vi "solar_log Banner Dialog.vi"() -> ()   [LabVIEW 2018]
doc: "This displays an error notification bar across the top of the primary monitor."
panel:
  in  "Close":bool
  in  "Error":string caption="Fault Summary:"
  # "ERROR"
  # "Click to Close"
  # "ERROR"
  # "Click to Close"
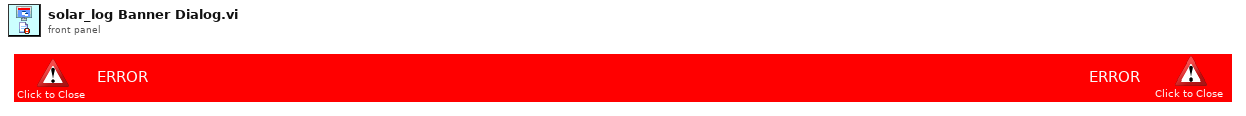
[diagram p1: front panel]
types:
  T1 = typedef "LVRectTypeDef.ctl" = cluster{"Left":i16, "Top":i16, "Right":i16, "Bottom":i16}
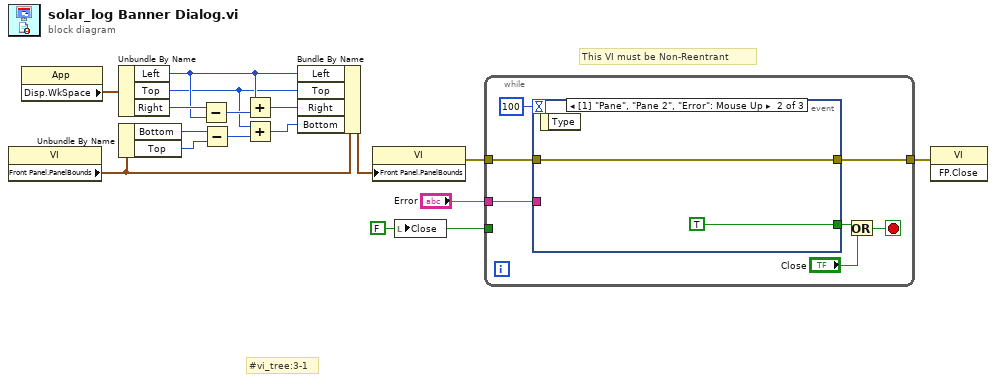
[diagram p0: block diagram]
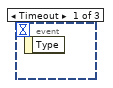
[diagram p2: hidden frame]
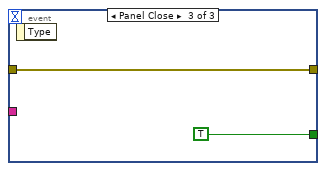
[diagram p3: hidden frame]
diagram:
  w1 = FALSE ("Close")
  # "#vi_tree:3-1"
  # "This VI must be Non-Reentrant"
  n1 = property class="VI"() -> ("Front Panel.PanelBounds"=w5:T1)  [unwired: 2 in, 2 out]
  n2 = property class="App"() -> ("Disp.WkSpace"=w15:T1)  [unwired: 2 in, 2 out]
  n3 = Unbundle By Name(w15) -> ("Left"=w7:i16, "Top"=w6:i16, "Right"=w8:i16)
  n4 = Unbundle By Name(w5) -> ("Bottom"=w4:i16, "Top"=w3:i16)
  n5 = Subtract(x=w8, y=w7) -> (x-y=w12:i16)
  n6 = Subtract(x=w4, y=w3) -> (x-y=w11:i16)
  n7 = Add(x=w7, y=w12) -> (x+y=w9:i16)
  n8 = Add(x=w6, y=w11) -> (x+y=w10:i16)
  n9 = Bundle By Name(cluster=w5, "Left"=w7, "Top"=w6, "Right"=w9, "Bottom"=w10) -> (w16:T1)
  n10 = property class="VI"("Front Panel.PanelBounds"=w16) -> (error out=w14:errorcluster)  [unwired: 2 in, 1 out]
  n11 = local write "Close"(w1) -> ()
  n12 = while {
    tunnel: w14 -> [w23]
    tunnel: "Error" -> [w22]
    tunnel: [w21] -> w2
    tunnel: w1 -> [_]
    stop <- w18 stop-if-true
    n13 = event shown="[1] \"Pane\", \"Pane 2\", \"Error\": Mouse Up" {
      selector: _ -> [_ _ _]
      dyn-events: _ -> [_ _ _]
      timeout: 100 -> [_ _ _]
      tunnel: w23 -> [_ w24 w26]
      tunnel: w22 -> [_ _ _]
      tunnel: [_ w24 w26] -> w21
      tunnel: [_ TRUE TRUE] -> w19
      event Timeout {
        n14 = event-data() -> ()  [unwired: 1 in, 1 out]
      }
      event "Error": Mouse Up {
        n15 = event-data() -> ()  [unwired: 1 in, 1 out]
      }
      event Panel Close {
        n16 = event-data() -> ()  [unwired: 1 in, 1 out]
      }
    }
    n17 = Or(x=w19, y="Close") -> (x .or. y?=w18:bool)
  }
  n18 = invoke class="VI" method="FP.Close"(error in=w2) -> ()  [unwired: 2 in, 3 out]
